vi "Write All.vi"(5 "Border Spacing":i16, 7 "Bounds":T2, 10 "Position":T1, 11 "(FPSZ)":refnum<class "FPSZ.lvclass">) -> (3 "(FPSZ) Out":refnum<class "FPSZ.lvclass">)   [LabVIEW 2023, in "FPSZ.lvclass"]
uses:
  FPSZ.lvclass
  <vilib>/Utility/miscctls.llb/LVBoundsTypeDef.ctl
  <vilib>/Utility/miscctls.llb/LVPositionTypeDef.ctl
  FPSZ.lvclass/FPSZ.ctl
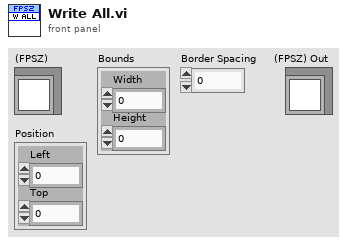
[diagram p1: front panel]
types:
  T1 = typedef "LVPositionTypeDef.ctl" = cluster{"Left":i32, "Top":i32}
  T2 = typedef "LVBoundsTypeDef.ctl" = cluster{"Width":u32, "Height":u32}
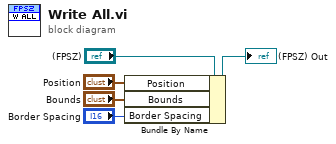
[diagram p0: block diagram]
diagram:
  n1 = Bundle By Name(cluster="(FPSZ)", "Position"="Position", "Bounds"="Bounds", "Border Spacing"="Border Spacing") -> (→"(FPSZ) Out":refnum<class "FPSZ.lvclass">)
